vi "Open Listening Server Reference.vi"(8 "error in (no error)":errorcluster, 11 "Generic Controller in":refnum<class "Generic Plugin.lvclass">) -> (0 "error out":errorcluster, 2 "vi reference":refnum<vi>, 3 "Generic Controller out":refnum<class "Generic Plugin.lvclass">)   [LabVIEW 2020, in "Generic Plugin.lvclass"]
uses:
  Generic Plugin.lvclass
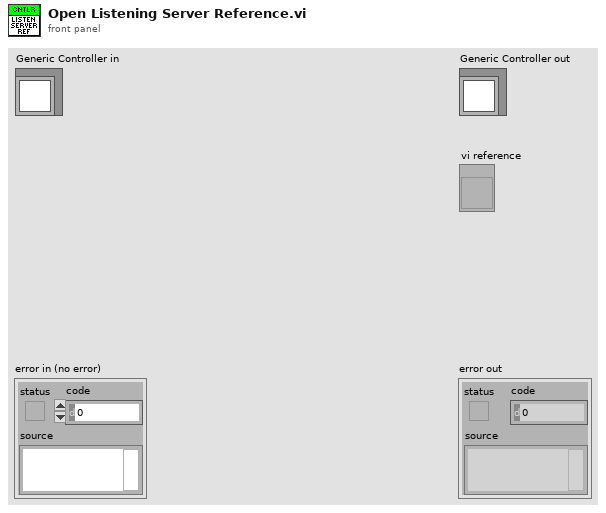
[diagram p1: front panel]
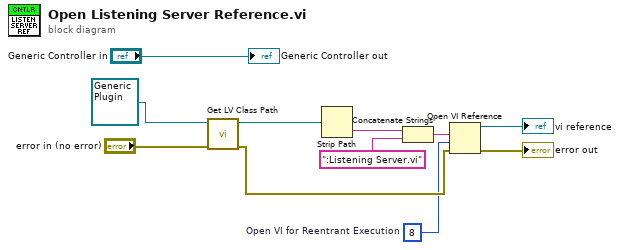
[diagram p0: block diagram]
diagram:
  w4 = 8  # Open VI for Reentrant Execution
  n1 = call <vilib>:"Get LV Class Path.vi"("error in (no error)"="error in (no error)", "object"=refnum<class "Generic Plugin.lvclass"> refnum ("Generic Controller in")) -> ("error out"=w9:errorcluster, "class path"=w5:path)  [unwired: 8 in]
  n2 = Strip Path(path=w5) -> (name=w6:string)  [unwired: 1 out]
  n3 = Concatenate Strings(w6, ":Listening Server.vi" ("string")) -> (w8:string)
  n4 = Open VI Reference(vi path=w8, options=w4, error in (no error)=w9) -> (vi reference=→"vi reference":refnum<vi>, error out=→"error out":errorcluster)  [unwired: 3 in]
  "Generic Controller out" <- "Generic Controller in"
